vi "Is Label Modified.vi"(9 "number of parameters":i32, 10 "initial index":i32, 11 "modified indices":i32[](array[numeric])) -> (2 "label modified":bool)   [LabVIEW 2020, in "AIM ARINC 429 Engine.lvlib" / "Implementation.lvlib" / "Tx Scheduled Labels Execution Unit.lvclass"]
doc: "Determines if a parameter has been modified based on the indices of modified elements from the <b>Values</b> array passed to Write to Hardware. The initial index should include the index of the disable parameter for the label."
uses:
  Tx Scheduled Labels Execution Unit.lvclass
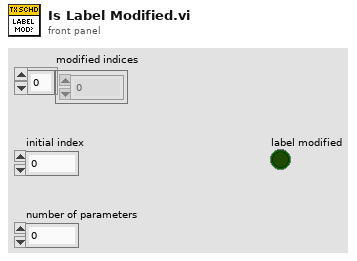
[diagram p1: front panel]
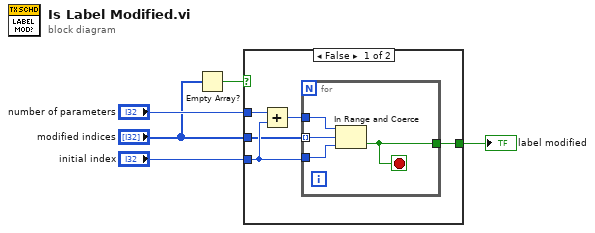
[diagram p0: block diagram]
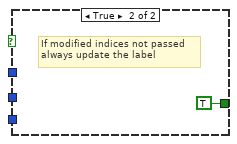
[diagram p2: hidden frame]
diagram:
  n1 = Empty Array?(array="modified indices") -> (empty?=w2:bool)
  n2 = case shown="False" w2 {
    tunnel: "initial index" -> [w9 _]
    tunnel: [w8 TRUE] -> w1
    tunnel: "number of parameters" -> [w7 _]
    tunnel: "modified indices" -> [w6 _]
    frame False {
      n3 = Add(x=w7, y=w9) -> (x+y=w10:i32)
      n4 = for {
        tunnel: w6 -> [w14] mode=indexing
        tunnel: w10 -> [w13]
        tunnel: w9 -> [w12]
        tunnel: [w11] -> w8
        stop <- w11 stop-if-true
        n5 = In Range and Coerce(upper limit=w13, x=w14, lower limit=w12) -> (In Range?=w11:bool)  [unwired: 1 out]
      }
    }
    frame True {
      # "If modified indices not passed\nalways update the label"
    }
  }
  "label modified" <- w1
